vi "Auton Action Monitor.vi"(8 "error in":errorcluster, 11 "occurrence":refnum<k4>) -> (0 "error out":errorcluster, 3 "Auton Monitor":T1)   [LabVIEW 2016, in "Auton Mode Base.lvclass"]
uses:
  Auton Mode Base.lvclass
  Auton Action Monitor Type.ctl
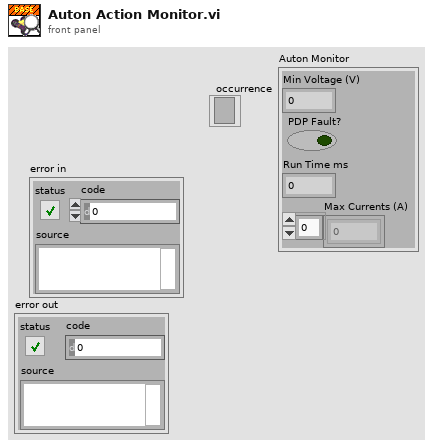
[diagram p1: front panel]
types:
  T1 = typedef "Auton Mode Base.lvclass/Auton Action Monitor Type.ctl" = cluster{"Min Voltage (V)":dbl, "PDP Fault?":bool, "Run Time ms":u32, "Max Currents (A)":dbl[]}
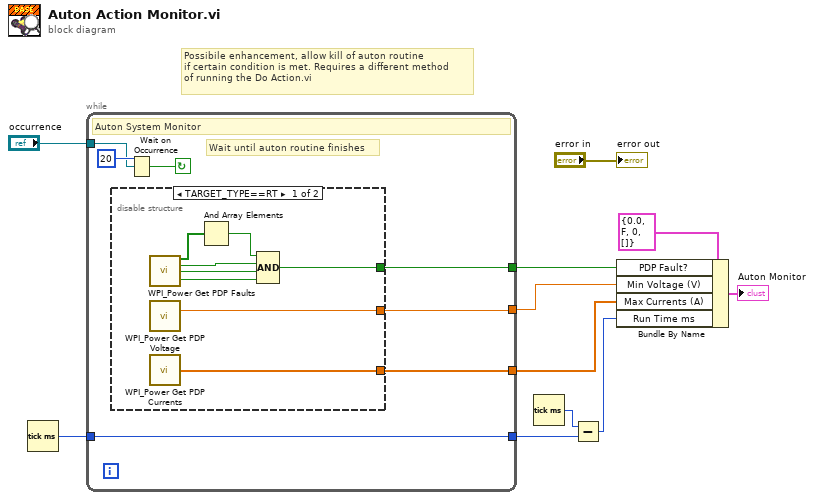
[diagram p0: block diagram]
diagram:
  # "Possibile enhancement, allow kill of auton routine\nif certain condition is met. Requires a different method\nof running the Do Action.vi"
  n1 = Tick Count (ms)() -> (millisecond timer value=w10:u32)
  n2 = while {
    tunnel: "occurrence" -> [w16]
    tunnel: [w15] -> w5
    tunnel: [w14] -> w4
    tunnel: [w13] -> w3
    tunnel: w10 -> [w12]
    tunnel: [w12] -> w8
    stop <- w17 continue-if-true
    # "Wait until auton routine finishes"
    # "Auton System Monitor"
    n3 = disable-structure shown="TARGET_TYPE==RT" {
      disable-tunnel: [w26 _] -> w15
      disable-tunnel: [w25 _] -> w14
      disable-tunnel: [w19 _] -> w13
      frame condition #0 (active) {
        n4 = call <vilib>:"WPI_Power Get PDP Faults.vi"() -> ("Current Faults"=w21:bool[], "Battery Voltage Fault"=w24:bool, "Temperature Fault"=w23:bool, "Hardware Fault"=w22:bool)  [unwired: 11 in, 1 out]
        n5 = call <vilib>:"WPI_Power Get PDP Voltage.vi"() -> ("voltage (V)"=w25:dbl)  [unwired: 14 in, 1 out]
        n6 = call <vilib>:"WPI_Power Get PDP Currents.vi"() -> ("all currents (A)"=w26:dbl[])  [unwired: 13 in, 2 out]
        n7 = And Array Elements(Boolean array=w21) -> (logical AND=w20:bool)
        n8 = Compound Arithmetic op=AND(w20, w24, w23, w22) -> (w19:bool)
      }
      frame condition #1 {
      }
    }
    n9 = Wait on Occurrence(2:w16, 3:20 ("ms timeout (-1)")) -> (0:w17:bool)  [unwired: 1 in]
  }
  n10 = Tick Count (ms)() -> (millisecond timer value=w9:u32)
  n11 = Subtract(x=w9, y=w8) -> (x-y=w6:u32)
  n12 = Bundle By Name(cluster=T1 {"Min Voltage (V)"=0.0, "PDP Fault?"=FALSE, "Run Time ms"=0, "Max Currents (A)"=[]}, "PDP Fault?"=w3, "Min Voltage (V)"=w4, "Max Currents (A)"=w5, "Run Time ms"=w6) -> (→"Auton Monitor":T1)
  "error out" <- "error in"
